vi "nanomsg_recvmsg.vi"(0 "socket in":refnum<class "nanomsg_socket.lvclass">, 1 "lenvec":i32[](array[numeric]), 2 "size":i32, 3 "error in":errorcluster, 4 "no block? (F)":bool) -> (5 "socket out":refnum<class "nanomsg_socket.lvclass">, 6 "parts":string[](array[string]), 7 "error out":errorcluster)   [LabVIEW 2014, in "nanomsg.lvlib" / "nanomsg_socket.lvclass"]
doc: "Receive a multi-component message from the socket. The incoming messages are returned as an array of strings, with one string for each message part.\n\nIf <b>no block?</b> is True, the function call will return immediately. \n\nOtherwise this call will block until <b>all</b> parts of the message are received, an error is raised, or the socket is closed."
uses:
  nanomsg_socket.lvclass
  nanomsg_socket.lvclass/nanomsg_socket.ctl
  <vilib>/Utility/error.llb/Error Cluster From Error Code.vi
  nanomsg.lvlib
panel:
  # "NN"
  # "labview"
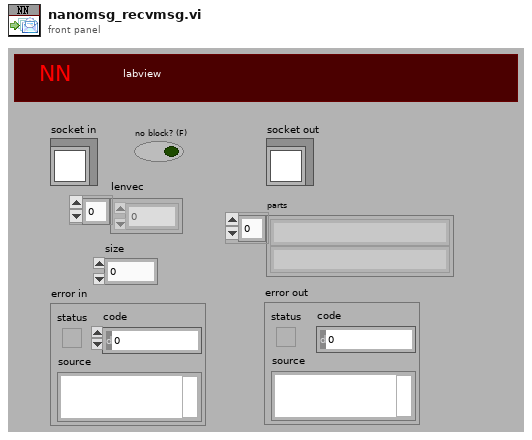
[diagram p1: front panel]
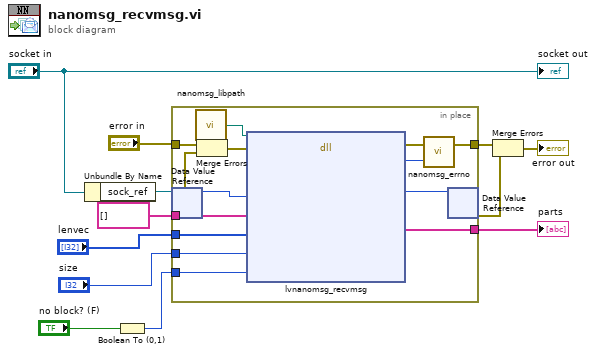
[diagram p0: block diagram]
diagram:
  n1 = Unbundle By Name("socket in") -> ("sock_ref"=w8:refnum<data-value>)
  n2 = Boolean To (0,1)(Boolean="no block? (F)") -> (0, 1=w1:i16)
  n3 = in-place {
    in-place-border: "error in" -> [w24]
    in-place-border: [w23] -> w11
    in-place-border: string[] [] ("parts") -> [w22]
    in-place-border: [w19] -> w7
    in-place-border: "lenvec" -> [w15]
    in-place-border: "size" -> [w14]
    in-place-border: w1 -> [w13]
    n4 = in-place-dvr #1(w8) -> (w21:u64, w16:errorcluster)
    n5 = call "nanomsg_libpath.vi"() -> ("path"=w18:path)
    n6 = Merge Errors(w24, w16) -> (w17:errorcluster)
    n7 = dll-call lib="?" fn="lvnanomsg_recvmsg" ("zmq_labview.dll:lvzmq_socket")(path in=w18, error in=w17, "sock_obj"=w21, "data"=w22, "lenvec"=w15, "size"=w14, "flags"=w13) -> (error out=w26:errorcluster, "return type"=w25:i32, "sock_obj"=w20:u64, "data"=w19:string[])  [unwired: 6 in, 1 out]
    n8 = call "nanomsg_errno.vi"("retval"=w25, "error in"=w26) -> ("error out"=w23:errorcluster)  [unwired: 1 out]
    n9 = in-place-dvr #1(w20) -> (w5:errorcluster)  [unwired: 1 out]
  }
  "parts" <- w7
  n10 = Merge Errors(w11, w5) -> (→"error out":errorcluster)
  "socket out" <- "socket in"
